vi "Main.vi"(10 "DAQ Type":enum16{"Hardware", "Simulation"}(ring), 11 "Module Admin":refnum<class "Delacor_lib_QMH_Module Admin.lvclass">) -> ()   [LabVIEW 2021, in "DAQ IO.lvlib"]
doc: "This template is based off of the Queued Message Handler design pattern and the Queued Message Handler project template that ships with LabVIEW.\n\nThe main difference is that the queue is private to this module and communication between modules is performed via Broadcast and Request events.\n\nRequest events are wrapped in public API methods and are handled in the Event Handling Loop (EHL) of this VI. Any module can register for Broadcast events sent by this module. The EHL generates messages based on user interface actions.\n\nThe Message Handling Loop (MHL) processes messages generated by the EHL, or by other messages. The messages are string values, so new messages can be added easily to the Message Cases case structure in the MHL. Each message cluster can also provide an optional value for Message Data, which is a variant that can be converted to whatever message-specific data is required.\n_____\nBased on DQMH Project Template 6.1.0.94."
uses:
  DAQ IO.lvlib
  <vilib>/Delacor/Delacor QMH/Libraries/Message Queue_class/Delacor_lib_QMH_Message Queue.lvclass
  Module Data--cluster.ctl
  <vilib>/Utility/miscctls.llb/LVPointTypeDef.ctl
  <vilib>/Utility/error.llb/Error Cluster From Error Code.vi
  <vilib>/ErrorRing/Error Ring.xnode
  <vilib>/Delacor/Delacor QMH/Libraries/Message Queue_class/Delacor_lib_QMH_Enqueue Message (Single).vi
  Stop Argument--cluster.ctl
  <vilib>/Delacor/Delacor QMH/Libraries/Module Admin_class/Delacor_lib_QMH_Module Admin.lvclass
  REQ Initialize DI (Reply Payload)--cluster.ctl
  REQ Initialize DI Argument--cluster.ctl
  Class/Abstract/Abstract.lvclass
  Class/PXI 6515/PXI 6515.lvclass
  REQ Initialize DO (Reply Payload)--cluster.ctl
  REQ Initialize DO Argument--cluster.ctl
  DO Name.ctl
  REQ Write DO Argument--cluster.ctl
  REQ Close DI Argument--cluster.ctl
  REQ Close DO Argument--cluster.ctl
  DI Channel Setting.ctl
  DO Channel Setting.ctl
  REQ Acq DI Argument--cluster.ctl
  C:/repository/common_ATE/Libraries/DAQ IO/Class/Abstract/Abstract.lvclass
  C:/repository/common_ATE/Libraries/DAQ IO/Class/PXI 6515/PXI 6515.lvclass
panel:
  out "DO  Setting":T1
  out "DI  Setting":T2
  in  "Acquire DI ?":bool
  out "error out":errorcluster
  out "Status":string
  in  "Simulate MHL Error":bool
  in  "Simulate EHL Error":bool
  # "Other QMH Modules communicate with this Module via its Public API (wrappers for its Request Events).\n\nThis Module communicates with other Modules via its Broadcast Events.\nAny module that wants to get these messages, just registers for this module's Broadcast events."
  # "This template is for the Delacor Modified Queued Message Handler design pattern.\n\nSee the block diagram for more information on how to use this template."
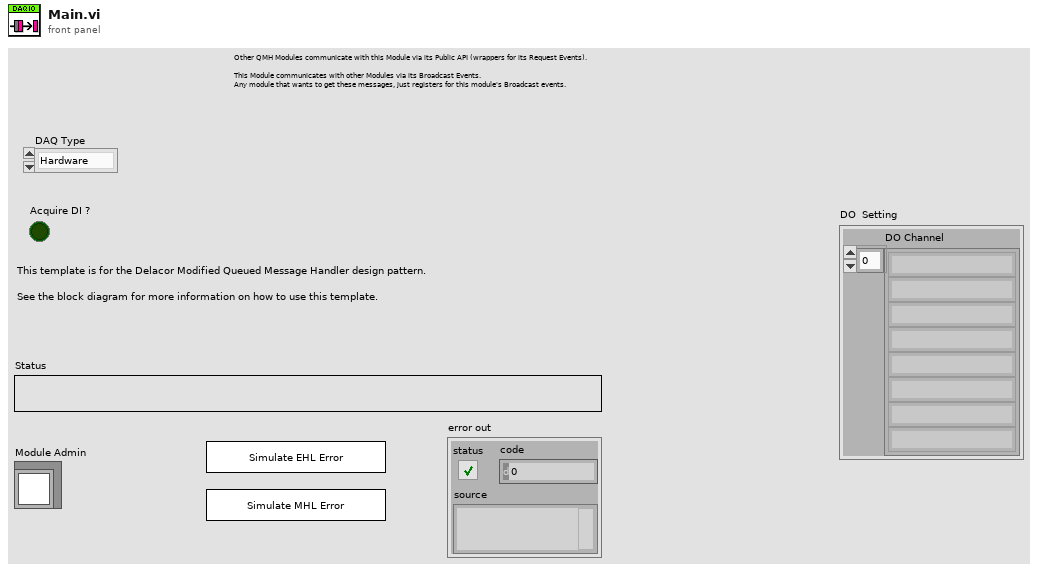
[diagram p1: front panel]
types:
  T1 = typedef "DAQ IO.lvlib/DO Channel Setting.ctl" = cluster{"DO Channel":string[]}
  T2 = typedef "DAQ IO.lvlib/DI Channel Setting.ctl" = cluster{"DI Channel":string[]}
  T3 = typedef "DAQ IO.lvlib/Module Data--cluster.ctl" = cluster{"Status":string, "Abstract.lvclass":refnum<class "Abstract.lvclass">, "DI Channel Setting":T2}
  T4 = typedef "DAQ IO.lvlib/Request Events--cluster.ctl" = cluster{"Stop Module":refnum<user-event>, "Show Panel":refnum<user-event>, "Hide Panel":refnum<user-event>, "Get Module Execution Status":refnum<user-event>, "Show Diagram":refnum<user-event>, "REQ Initialize DI":refnum<user-event>, "REQ Initialize DO":refnum<user-event>, "REQ Write DO":refnum<user-event>, "REQ Close DI":refnum<user-event>, "REQ Close DO":refnum<user-event>, "REQ Acq DI":refnum<user-event>}
  T5 = enum32{"invalid lock state", "Not Locked", "Locked (No Password)", "Password-protected"}
  T6 = typedef "DAQ IO.lvlib/Stop Argument--cluster.ctl" = cluster{"Origin":string, "Exit via Stop Module Req?":bool, "Wait for Module to stop?":bool}
  T7 = typedef "DAQ IO.lvlib/REQ Initialize DI Argument--cluster.ctl" = cluster{"Wait Notifier":refnum<notifier>, "wait for reply":bool, "DI Channel Setting":T2}
  T8 = typedef "DAQ IO.lvlib/REQ Initialize DO Argument--cluster.ctl" = cluster{"Wait Notifier":refnum<notifier>, "wait for reply":bool, "DO Channel Setting":T1}
  T9 = typedef "DAQ IO.lvlib/REQ Write DO Argument--cluster.ctl" = cluster{"DO Name":T10, "DO Value":bool[]}
  T10 = typedef "DAQ IO.lvlib/DO Name.ctl" = enum16{"Emg", "Start", "Stop", "Retry"}
  T11 = typedef "DAQ IO.lvlib/REQ Close DI Argument--cluster.ctl" = cluster{"Boolean":bool}
  T12 = typedef "DAQ IO.lvlib/REQ Close DO Argument--cluster.ctl" = cluster{"Boolean":bool}
  T13 = typedef "DAQ IO.lvlib/REQ Acq DI Argument--cluster.ctl" = cluster{"Acq DI":bool}
  T14 = typedef "LVPointTypeDef.ctl" = cluster{"Horizontal":i16, "Vertical":i16}
  T15 = enum32{"Invalid", "Standard", "Closed", "Hidden", "Minimized", "Maximized"}
  T16 = typedef "DAQ IO.lvlib/REQ Initialize DI (Reply Payload)--cluster.ctl" = cluster{"Connect?":bool, "error":errorcluster}
  T17 = typedef "DAQ IO.lvlib/REQ Initialize DO (Reply Payload)--cluster.ctl" = cluster{"Connect?":bool, "error":errorcluster}
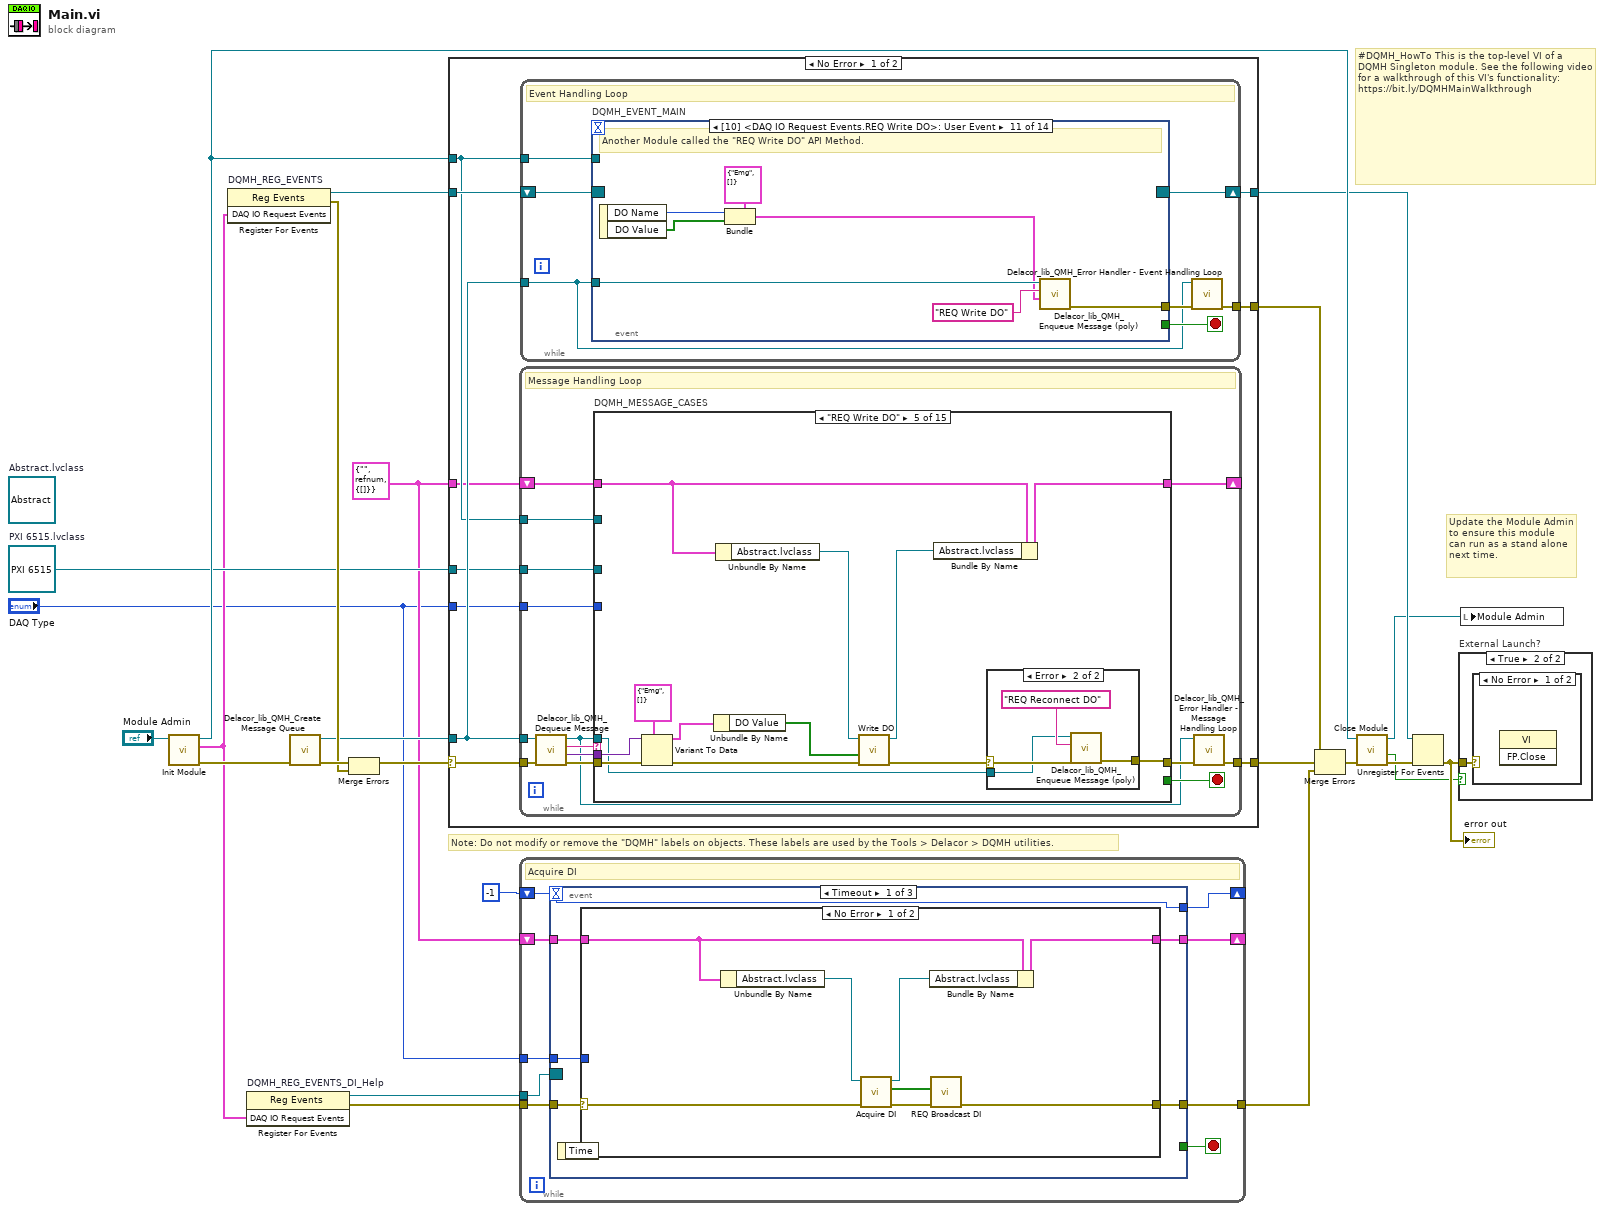
[diagram p0: block diagram]
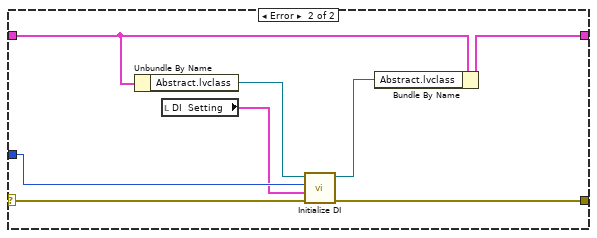
[diagram p2: hidden frame]
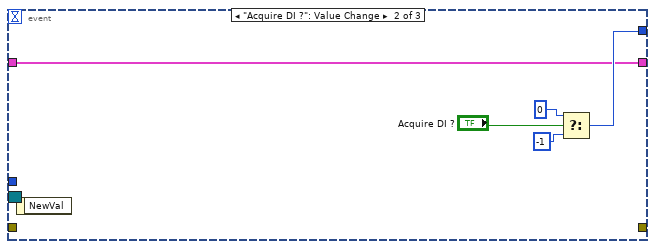
[diagram p3: hidden frame]
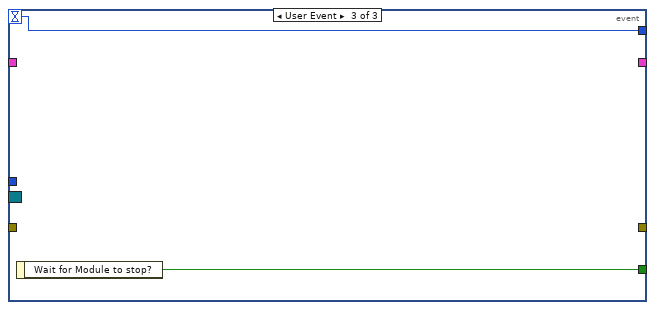
[diagram p4: hidden frame]
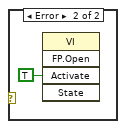
[diagram p6: hidden frame]
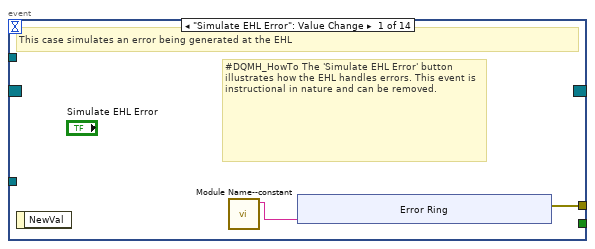
[diagram p7: hidden frame]
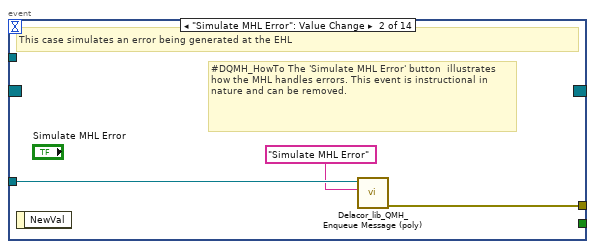
[diagram p8: hidden frame]
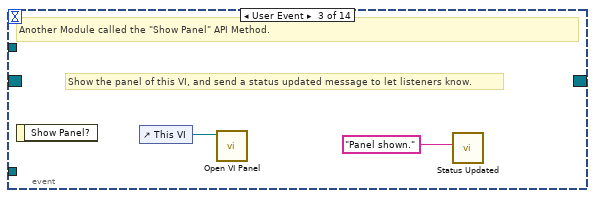
[diagram p9: hidden frame]
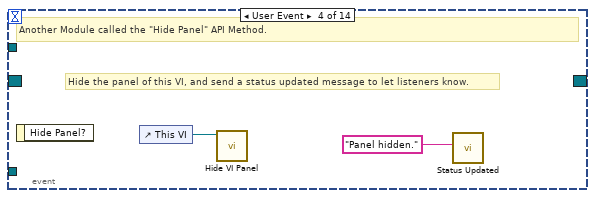
[diagram p10: hidden frame]
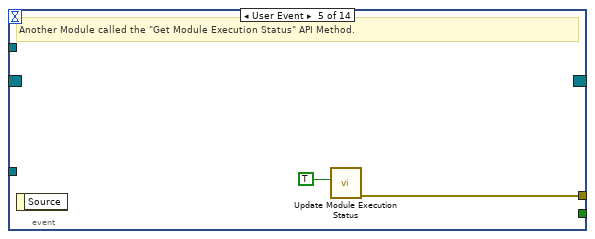
[diagram p11: hidden frame]
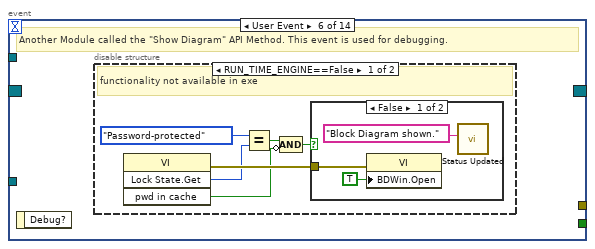
[diagram p12: hidden frame]
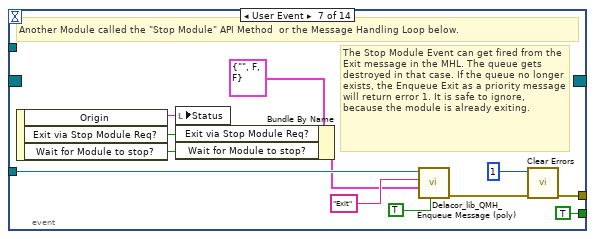
[diagram p15: hidden frame]
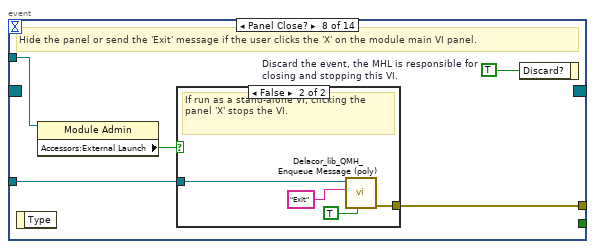
[diagram p16: hidden frame]
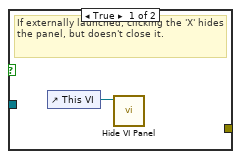
[diagram p17: hidden frame]
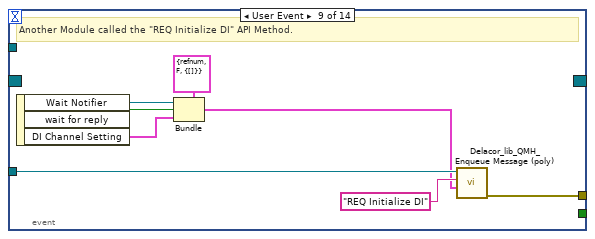
[diagram p18: hidden frame]
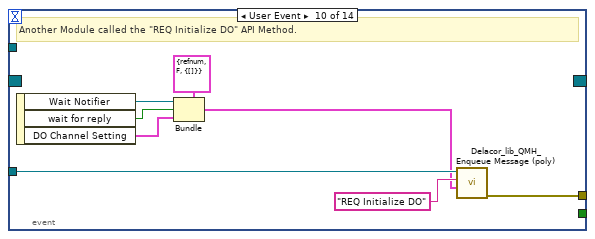
[diagram p19: hidden frame]
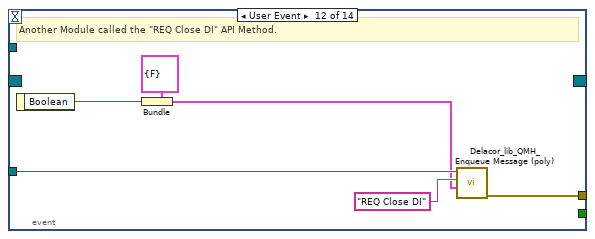
[diagram p20: hidden frame]
diagram:
  w4 = T3 {"Status"="", "Abstract.lvclass"=refnum, "DI Channel Setting"={"DI Channel"=[]}} ("Data Cluster")
  w9 = refnum<class "PXI 6515.lvclass"> refnum  # PXI 6515.lvclass
  (unwired) refnum<class "Abstract.lvclass"> refnum  # Abstract.lvclass
  # "#DQMH_HowTo This is the top-level VI of a DQMH Singleton module. See the following video for a walkthrough of this VI's functionality: https://bit.ly/DQMHMainWalkthrough"
  # "Note: Do not modify or remove the \"DQMH\" labels on objects. These labels are used by the Tools > Delacor > DQMH utilities."
  # "Update the Module Admin to ensure this module can run as a stand alone next time."
  n1 = call "Init Module.vi"("Singleton Module Admin in"="Module Admin") -> ("error out"=w23:errorcluster, "DAQ IO Request Events"=w8:T4, "Singleton Module Admin out"=w16:refnum<class "Delacor_lib_QMH_Module Admin.lvclass">)  [unwired: 8 in]
  n2 = register-events "DQMH_REG_EVENTS"(w8) -> (reference out=w14:refnum<event-registration>, error out=w17:errorcluster)  [unwired: 2 in]
  n3 = register-events "DQMH_REG_EVENTS_DI_Help"(w8) -> (reference out=w7:refnum<event-registration>, error out=w6:errorcluster)  [unwired: 2 in]
  n4 = call <vilib>:"Delacor_lib_QMH_Create Message Queue.vi"("error in"=w23) -> ("error out"=w19:errorcluster, "Message Queue"=w13:refnum<class "Delacor_lib_QMH_Message Queue.lvclass">)  [unwired: 9 in]
  n5 = Merge Errors(w19, w17) -> (w18:errorcluster)
  n6 = case shown="No Error" w18 {
    selector: w18 -> [w32 w327]
    tunnel: [w34 w326] -> w24
    tunnel: [w31 w332] -> w15
    tunnel: w14 -> [w30 w332]
    tunnel: w13 -> [w29 w325]
    tunnel: [w33 _] -> w3
    tunnel: w16 -> [w28 w328]
    tunnel: w9 -> [w27 _]
    tunnel: "DAQ Type" -> [w26 _]
    tunnel: w4 -> [w25 _]
    frame No Error {
      n7 = while {
        tunnel: w29 -> [w136]
        shift-right: [w140] -> _
        shift-left: w25 -> [w141]
        tunnel: w32 -> [w144]
        tunnel: [w142] -> w34
        tunnel: w28 -> [w134]
        tunnel: w27 -> [w133]
        tunnel: w26 -> [w132]
        stop <- w139 stop-if-true
        # "Message Handling Loop"
        n8 = call-dynamic "Delacor_lib_QMH_Dequeue Message.vi"("error in"=w144, "Message Queue in"=w136) -> ("error out"=w143:errorcluster, "Message Data"=w137:variant, "Message"=w138:string, "Message Queue out"=w135:refnum<class "Delacor_lib_QMH_Message Queue.lvclass">)  [unwired: 6 in]
        n9 = case "DQMH_MESSAGE_CASES" shown="\"REQ Write DO\"" w138 {
          selector: w138 -> [_ _ _ _ _ _ _ _ _ _ _ _ _ _ w312]
          tunnel: w135 -> [_ _ _ _ w209 _ _ w251 _ _ _ _ w282 w304 _]
          tunnel: w143 -> [w164 w168 w186 w206 w221 w236 w246 w253 w262 w265 w267 w272 w289 w310 w314]
          tunnel: [w162 w168 w175 w195 w210 w231 w241 w252 w255 w264 w267 w271 w285 w307 w315] -> w145
          tunnel: w141 -> [w153 w167 w172 w191 w216 w230 w240 w254 w261 w263 w266 w269 w284 w303 w313]
          tunnel: [w152 w167 w176 w197 w214 w228 w238 w254 w261 w263 w266 w269 w284 w303 w313] -> w140
          tunnel: [_ _ _ _ _ _ _ _ _ _ _ _ _ w302 _] -> w139
          tunnel: w137 -> [_ _ w185 w205 w220 w235 w245 _ w260 _ _ _ w283 w301 _]
          tunnel: w134 -> [w154 _ _ _ _ _ _ _ _ _ _ _ w281 w296 _]
          tunnel: w133 -> [w146 _ _ _ _ _ _ _ _ _ _ _ _ _ _]
          tunnel: w132 -> [_ _ w177 w192 _ _ _ _ _ _ _ _ _ _ _]
          frame "Initialize" {
            w148 = "Initial Message" ("Initial Message")
            # "Initialize - Any operation that needs to be done before the module can receive messages. Synchronize Caller Events.vi will inform Start Module.vi that the module has launched and is ready to receive messages. Module Did Init.vi will broadcast that the module initialized."
            n10 = call "Synchronize Caller Events.vi"("error in (no error)"=w164, "Singleton Module Admin in"=w154) -> ("error out"=w163:errorcluster, "Singleton Module Admin out"=w149:refnum<class "Delacor_lib_QMH_Module Admin.lvclass">)  [unwired: 8 in]
            n11 = property class="Module Admin"(reference=w149) -> ("Accessors:External Launch"=w158:bool)  [unwired: 1 in, 2 out]
            n12 = Select(t=T15."Hidden" ("State"), s=w158, f=T15."Standard" ("State")) -> (s? t:f=w155:T15)
            n13 = call "Module Name--constant.vi"() -> ("Module Name"=w161:string)  [unwired: 11 in]
            n14 = property class="VI"("Front Panel.Title"=w161) -> (reference out=w160:refnum<vi>, error out=w166:errorcluster)  [unwired: 2 in]
            n15 = call "Module Name--constant.vi"() -> ("Module Name"=w150:string)  [unwired: 11 in]
            n16 = Bundle By Name(cluster=w153, "Status"=w148, "Abstract.lvclass"=w146) -> (w152:T3)
            n17 = invoke class="VI" method="FP.Open"(reference=w160, error in=w166, "State"=w155) -> (reference out=w159:refnum<vi>, error out=w165:errorcluster)  [unwired: 2 in, 3 out]
            n18 = call "Module Did Init.vi"("error in (no error)"=w163, "Initialized?"=TRUE, "Origin"=w150) -> ("error out"=w162:errorcluster)  [unwired: 8 in]
            n19 = invoke class="VI" method="FP.Center"(reference=w159, error in=w165) -> ()  [unwired: 1 in, 3 out]
            n20 = property on="Pane" class="Pane"("Origin"=T14 {"Horizontal"=0, "Vertical"=0}) -> ()  [unwired: 2 in, 2 out]
            "Status" <- w148
          }
          frame "---Module Specific---" {
            # "Separator -- The following cases handle messages specific to this Module."
          }
          frame "REQ Initialize DI" {
            n21 = Variant To Data(error in=w186, type=T7 {"Wait Notifier"=refnum, "wait for reply"=FALSE, "DI Channel Setting"={"DI Channel"=[]}} ("REQ Initialize DI Argument"), Variant=w185) -> (data=w183:T7, error out=w178:errorcluster)
            n22 = Unbundle By Name(w183) -> ("Wait Notifier"=w182:refnum<notifier>, "wait for reply"=w181:bool, "DI Channel Setting"=w169:T2)
            "DI  Setting" <- w169
            n23 = Unbundle By Name(w172) -> ("Abstract.lvclass"=w171:refnum<class "Abstract.lvclass">)
            n24 = call-dynamic "Initialize DI.vi"("error in (no error)"=w178, "DI Channel Setting"=w169, "DAQ Type"=w177, "Abstract in"=w171) -> ("error out"=w175:errorcluster, "Abstract out"=w170:refnum<class "Abstract.lvclass">)  [unwired: 6 in]
            n25 = Unbundle By Name(w175) -> ("status"=w174:bool)
            n26 = Bundle By Name(cluster=w172, "Abstract.lvclass"=w170) -> (w176:T3)
            n27 = Not(x=w174) -> (.not. x?=w173:bool)
            n28 = Bundle By Name(cluster=T16 {"Connect?"=FALSE, "error"={"status"=FALSE, "code"=0, "source"=""}} ("REQ Initialize DI (Reply Payload)"), "Connect?"=w173) -> (w180:T16)
            n29 = case shown="True" w181 {
              tunnel: w182 -> [_ w188]
              tunnel: w180 -> [_ w187]
              frame False {
              }
              frame True {
                n30 = Send Notification(notification=w187, notifier=w188) -> ()  [unwired: 1 in, 2 out]
              }
            }
          }
          frame "REQ Initialize DO" {
            n31 = Variant To Data(error in=w206, type=T8 {"Wait Notifier"=refnum, "wait for reply"=FALSE, "DO Channel Setting"={"DO Channel"=[]}} ("REQ Initialize DO Argument"), Variant=w205) -> (data=w203:T8, error out=w198:errorcluster)
            n32 = Unbundle By Name(w191) -> ("Abstract.lvclass"=w190:refnum<class "Abstract.lvclass">)
            n33 = Unbundle By Name(w203) -> ("Wait Notifier"=w202:refnum<notifier>, "wait for reply"=w201:bool, "DO Channel Setting"=w189:T1)
            "DO  Setting" <- w189
            n34 = call-dynamic "Initialize DO.vi"("error in (no error)"=w198, "DO Channel Setting"=w189, "DAQ Type"=w192, "Abstract in"=w190) -> ("error out"=w195:errorcluster, "Abstract out"=w196:refnum<class "Abstract.lvclass">)  [unwired: 6 in]
            n35 = Unbundle By Name(w195) -> ("status"=w194:bool)
            n36 = Bundle By Name(cluster=w191, "Abstract.lvclass"=w196) -> (w197:T3)
            n37 = Not(x=w194) -> (.not. x?=w193:bool)
            n38 = Bundle By Name(cluster=T17 {"Connect?"=FALSE, "error"={"status"=FALSE, "code"=0, "source"=""}} ("REQ Initialize DO (Reply Payload)"), "Connect?"=w193) -> (w200:T17)
            n39 = case shown="True" w201 {
              tunnel: w202 -> [_ w208]
              tunnel: w200 -> [_ w207]
              frame False {
              }
              frame True {
                n40 = Send Notification(notification=w207, notifier=w208) -> ()  [unwired: 1 in, 2 out]
              }
            }
          }
          frame "REQ Write DO" {
            n41 = Variant To Data(error in=w221, type=T9 {"DO Name"=enum."Emg", "DO Value"=[]} ("REQ Write DO Argument"), Variant=w220) -> (data=w218:T9, error out=w217:errorcluster)
            n42 = Unbundle By Name(w218) -> ("DO Value"=w212:bool[])
            n43 = Unbundle By Name(w216) -> ("Abstract.lvclass"=w215:refnum<class "Abstract.lvclass">)
            n44 = call-dynamic "Write DO.vi"("error in (no error)"=w217, "DO Value"=w212, "Abstract in"=w215) -> ("error out"=w211:errorcluster, "Abstract out"=w213:refnum<class "Abstract.lvclass">)  [unwired: 7 in]
            n45 = Bundle By Name(cluster=w216, "Abstract.lvclass"=w213) -> (w214:T3)
            n46 = case shown="Error" w211 {
              selector: w211 -> [w222 w225]
              tunnel: [w222 w224] -> w210
              tunnel: w209 -> [_ w223]
              frame No Error {
              }
              frame Error {
                n47 = call-poly <vilib>:"Delacor_lib_QMH_Enqueue Message (poly).vi"("error in"=w225, "Message"="REQ Reconnect DO", "Message Queue in"=w223) -> ("error out"=w224:errorcluster)  [unwired: 7 in, 1 out]
              }
            }
          }
          frame "REQ Close DI" {
            n48 = Variant To Data(error in=w236, type=T11 {"Boolean"=FALSE} ("REQ Close DI Argument"), Variant=w235) -> (data=w233:T11, error out=w232:errorcluster)
            n49 = Unbundle By Name(w233) -> ()  [unwired: 1 out]
            n50 = Unbundle By Name(w230) -> ("Abstract.lvclass"=w229:refnum<class "Abstract.lvclass">)
            n51 = call-dynamic "Close DI Ref.vi"("error in (no error)"=w232, "Abstract in"=w229) -> ("error out"=w231:errorcluster, "Abstract out"=w227:refnum<class "Abstract.lvclass">)  [unwired: 8 in]
            n52 = Bundle By Name(cluster=w230, "Abstract.lvclass"=w227) -> (w228:T3)
          }
          frame "REQ Close DO" {
            n53 = Variant To Data(error in=w246, type=T12 {"Boolean"=FALSE} ("REQ Close DO Argument"), Variant=w245) -> (data=w243:T12, error out=w242:errorcluster)
            n54 = Unbundle By Name(w243) -> ()  [unwired: 1 out]
            n55 = Unbundle By Name(w240) -> ("Abstract.lvclass"=w239:refnum<class "Abstract.lvclass">)
            n56 = call-dynamic "Close DO Ref.vi"("error in (no error)"=w242, "Abstract in"=w239) -> ("error out"=w241:errorcluster, "Abstract out"=w237:refnum<class "Abstract.lvclass">)  [unwired: 8 in]
            n57 = Bundle By Name(cluster=w240, "Abstract.lvclass"=w237) -> (w238:T3)
          }
          frame "REQ Reconnect DO" {
            # "Duplicate this frame when creating new messages.  Change this comment in the duplicated frame to describe this message."
            n58 = local read "DO  Setting"() -> (w248:T1)
            n59 = Bundle By Name(cluster=T8 {"Wait Notifier"=refnum, "wait for reply"=FALSE, "DO Channel Setting"={"DO Channel"=[]}} ("REQ Initialize DO Argument"), "DO Channel Setting"=w248) -> (w247:T8)
            n60 = call-poly <vilib>:"Delacor_lib_QMH_Enqueue Message (poly).vi"("error in"=w253, "Message Data"=w247, "Message"="REQ Initialize DO" ("String"), "Message Queue in"=w251) -> ("error out"=w252:errorcluster)  [unwired: 6 in, 1 out]
          }
          frame "REQ Acq DI" {
            n61 = Variant To Data(error in=w262, type=T13 {"Acq DI"=FALSE} ("REQ Acq DI Argument"), Variant=w260) -> (data=w258:T13, error out=w257:errorcluster)
            n62 = Unbundle By Name(w258) -> ("Acq DI"=w256:bool)
            n63 = property on="Acquire DI ?" class="Bool (strict)"(error in=w257, "Val(Sgnl)"=w256) -> (error out=w255:errorcluster)  [unwired: 1 in, 1 out]
          }
          frame "---Copy This Frame---" {
            # "Duplicate this frame when creating new messages.  Change this comment in the duplicated frame to describe this message."
            n64 = Merge Errors(w265) -> (w264:errorcluster)
          }
          frame "---Exit and Error Handling---" {
            # "Separator - The following cases handle errors and exit messages."
          }
          frame "Simulate MHL Error" {
            # "#DQMH_HowTo The 'Simulate MHL Error' button  illustrates how the MHL handles errors. This event is instructional in nature and can be removed."
            # "Simulate an error occurring at the MHL"
            n65 = call "Module Name--constant.vi"() -> ("Module Name"=w268:string)  [unwired: 11 in]
            n66 = xnode "Error Ring"("parameter 0"=w268) -> ("error out"=w270:errorcluster)
            n67 = Merge Errors(w272, w270) -> (w271:errorcluster)
          }
          frame "Error" {
            # "#CodeRecommended - If you ever change the name of this \"Error\" message, you'll need to update the name in the Check Loop Error.vi as well."
            # "#CodeRecommended - If the module is running in standalone mode (External Launch = FALSE), this code will pop up an error dialog and call the 'Exit' message if an error occurs. Add more fine-grained error handling here."
            # "Error - Check the error message data and respond accordingly. This message is sent by the \"Error Handler\" VIs at the end of each loop in this application."
            n68 = property class="Module Admin"(reference=w281) -> ("Accessors:External Launch"=w280:bool)  [unwired: 1 in, 2 out]
            n69 = Variant To Data(error in=w289, type=errorcluster {"status"=FALSE, "code"=0, "source"=""} ("error constant"), Variant=w283) -> (data=w290:errorcluster, error out=w287:errorcluster)
            n70 = call "Error Reported.vi"("Error"=w290) -> ()  [unwired: 10 in, 1 out]
            n71 = case shown="False" w280 {
              tunnel: [w295 _] -> w286
              tunnel: w282 -> [w293 _]
              tunnel: w290 -> [w294 _]
              frame False {
                (unwired) "Exit"
                n72 = call <vilib>:"Simple Error Handler.vi"("error in (no error)"=w294) -> ()  [unwired: 4 in, 5 out]
                n73 = call-poly <vilib>:"Delacor_lib_QMH_Enqueue Message (poly).vi"("Priority Message? (F)"=TRUE, "Message"="REQ Reconnect", "Message Queue in"=w293) -> ("error out"=w295:errorcluster)  [unwired: 7 in, 1 out]
              }
              frame True {
                # "If the module was launched externally, calling the Error Reported broadcast VI is the only action performed by the \"Error\" message. The module's caller can then process the error appropriately."
              }
            }
            n74 = Merge Errors(w287, w286) -> (w285:errorcluster)
            n75 = local write "error out"(w285) -> ()
          }
          frame "Exit" {
            w300 = 91  # 91: not all Exit messages will have an argument
            w302 = TRUE  # Stop the VI
            # "Release the message queue reference"
            # "#CodeNeeded - Add any required cleanup code here"
            # "Exit - Exit the application."
            n76 = Variant To Data(error in=w310, type=T6 {"Origin"="", "Exit via Stop Module Req?"=FALSE, "Wait for Module to stop?"=FALSE} ("Stop Argument"), Variant=w301) -> (data=w298:T6, error out=w306:errorcluster)
            n77 = call <vilib>:"Clear Errors.vi"("error in (no error)"=w306, "specific error code to clear (0: all)"=w300) -> ("error out"=w309:errorcluster)  [unwired: 4 in, 1 out]
            n78 = control-ref of="This VI"() -> (w297:refnum<vi>)
            n79 = call-dynamic "Delacor_lib_QMH_Release Message Queue.vi"("error in"=w309, "Message Queue"=w304) -> ("error out"=w308:errorcluster)  [unwired: 9 in]
            n80 = call "Handle Exit.vi"("Stop Argument"=w298, "Admin in"=w296, "VI reference"=w297) -> ("error out"=w305:errorcluster)  [unwired: 7 in, 1 out]
            n81 = Merge Errors(w308, w305) -> (w307:errorcluster)
          }
          frame Default {
            # "'Default' case only runs if there is a message that isn't defined in any of the other cases.  Output a programming error."
            n82 = call "Module Name--constant.vi"() -> ("Module Name"=w311:string)  [unwired: 11 in]
            n83 = xnode "Error Ring"("parameter 0"=w312, "parameter 1"=w311) -> ("error out"=w316:errorcluster)
            n84 = Merge Errors(w314, w316) -> (w315:errorcluster)
          }
        }
        n85 = call-dynamic "Delacor_lib_QMH_Error Handler - Message Handling Loop.vi"("error in"=w145, "Message Queue in"=w135) -> ("dup error in"=w142:errorcluster)  [unwired: 8 in, 1 out]
      }
      n86 = while {
        tunnel: w29 -> [w35]
        shift-right: [w38] -> w31
        shift-left: w30 -> [w39]
        tunnel: [w40] -> w33
        tunnel: w28 -> [w36]
        stop <- w37 stop-if-true
        # "Event Handling Loop"
        n87 = event "DQMH_EVENT_MAIN" shown="[10] <DAQ IO Request Events.REQ Write DO>: User Event" {
          selector: w39 -> [_ _ _ _ _ _ _ _ _ _ _ _ _ _]
          dyn-events: [_ _ _ _ _ _ _ _ _ _ _ _ _ _] -> w38
          timeout: _ -> [_ _ _ _ _ _ _ _ _ _ _ _ _ _]
          tunnel: [_ _ _ _ _ _ TRUE ("Discard?") _ _ _ _ _ _ _] -> w37
          tunnel: w35 -> [_ w52 _ _ _ _ w76 w83 w98 w106 w113 w119 w125 w131]
          tunnel: [w43 w53 _ _ w59 _ w79 w85 w94 w100 w107 w114 w120 w126] -> w41
          tunnel: w36 -> [_ _ _ _ _ _ _ w82 _ _ _ _ _ _]
          event "Simulate EHL Error": Value Change {
            # "#DQMH_HowTo The 'Simulate EHL Error' button  illustrates how the EHL handles errors. This event is instructional in nature and can be removed."
            # "This case simulates an error being generated at the EHL"
            n88 = event-data() -> ()  [unwired: 1 in, 1 out]
            n89 = call "Module Name--constant.vi"() -> ("Module Name"=w42:string)  [unwired: 11 in]
            n90 = xnode "Error Ring"("parameter 0"=w42) -> ("error out"=w43:errorcluster)
          }
          event "Simulate MHL Error": Value Change {
            # "#DQMH_HowTo The 'Simulate MHL Error' button  illustrates how the MHL handles errors. This event is instructional in nature and can be removed."
            # "This case simulates an error being generated at the EHL"
            n91 = event-data() -> ()  [unwired: 1 in, 1 out]
            n92 = call-poly <vilib>:"Delacor_lib_QMH_Enqueue Message (poly).vi"("Message"="Simulate MHL Error", "Message Queue in"=w52) -> ("error out"=w53:errorcluster)  [unwired: 8 in, 1 out]
          }
          event User Event {
            # "Show the panel of this VI, and send a status updated message to let listeners know."
            # "Another Module called the \"Show Panel\" API Method."
            n93 = event-data() -> ()  [unwired: 1 in, 1 out]
            n94 = control-ref of="This VI"() -> (w55:refnum<vi>)
            n95 = call "Open VI Panel.vi"("VI"=w55) -> ()  [unwired: 10 in, 1 out]
            n96 = call "Status Updated.vi"("Status"="Panel shown." ("format string")) -> ()  [unwired: 10 in, 1 out]
          }
          event User Event {
            # "Hide the panel of this VI, and send a status updated message to let listeners know."
            # "Another Module called the \"Hide Panel\" API Method."
            n97 = event-data() -> ()  [unwired: 1 in, 1 out]
            n98 = control-ref of="This VI"() -> (w57:refnum<vi>)
            n99 = call "Hide VI Panel.vi"("VI"=w57) -> ()  [unwired: 10 in, 1 out]
            n100 = call "Status Updated.vi"("Status"="Panel hidden." ("format string")) -> ()  [unwired: 10 in, 1 out]
          }
          event User Event {
            # "Another Module called the \"Get Module Execution Status\" API Method."
            n101 = event-data() -> ()  [unwired: 1 in, 1 out]
            n102 = call "Update Module Execution Status.vi"("Running?"=TRUE) -> ("error out"=w59:errorcluster)  [unwired: 10 in]
          }
          event User Event {
            # "Another Module called the \"Show Diagram\" API Method. This event is used for debugging."
            n103 = event-data() -> ()  [unwired: 1 in, 1 out]
            n104 = disable-structure shown="RUN_TIME_ENGINE==False" {
              frame condition #0 (active) {
                # "functionality not available in exe"
                n105 = invoke class="VI" method="Lock State.Get"() -> (error out=w65:errorcluster, "Get Lock State"=w64:T5, "pwd in cache"=w61:bool)  [unwired: 4 in, 1 out]
                n106 = Equal?(x=T5."Password-protected", y=w64) -> (x = y?=w62:bool)
                n107 = Compound Arithmetic op=AND(w62, invert w61) -> (w60:bool)
                n108 = case shown="False" w60 {
                  tunnel: w65 -> [w68 _]
                  frame False {
                    n109 = property class="VI"(error in=w68, "BDWin.Open"=TRUE ("Block Diagram Window:Open")) -> ()  [unwired: 1 in, 2 out]
                    n110 = call "Status Updated.vi"("Status"="Block Diagram shown." ("format string")) -> ()  [unwired: 10 in, 1 out]
                  }
                  frame True {
                    # "Password-protected VI, and the password is not in the cache. Do not show the diagram."
                  }
                }
              }
              frame condition #1 {
              }
            }
          }
          event User Event {
            # "The Stop Module Event can get fired from the Exit message in the MHL. The queue gets destroyed in that case. If the queue no longer exists, the Enqueue Exit as a priority message will return error 1. It is safe to ignore, because the module is already exiting."
            # "Another Module called the \"Stop Module\" API Method  or the Message Handling Loop below."
            n111 = event-data() -> ("Origin"=w75:string, "Exit via Stop Module Req?"=w71:bool, "Wait for Module to stop?"=w70:bool)  [unwired: 1 in]
            n112 = local write "Status"(w75) -> ()
            n113 = Bundle By Name(cluster=T6 {"Origin"="", "Exit via Stop Module Req?"=FALSE, "Wait for Module to stop?"=FALSE} ("Stop Argument"), "Exit via Stop Module Req?"=w71, "Wait for Module to stop?"=w70) -> (w69:T6)
            n114 = call-poly <vilib>:"Delacor_lib_QMH_Enqueue Message (poly).vi"("Priority Message? (F)"=TRUE, "Message Data"=w69, "Message"="Exit", "Message Queue in"=w76) -> ("error out"=w80:errorcluster)  [unwired: 6 in, 1 out]
            n115 = call <vilib>:"Clear Errors.vi"("error in (no error)"=w80, "specific error code to clear (0: all)"=1) -> ("error out"=w79:errorcluster)  [unwired: 4 in, 1 out]
          }
          event Panel Close? {
            w84 = TRUE  # Discard the event, the MHL is responsible for closing and stopping this VI.
            # "Hide the panel or send the 'Exit' message if the user clicks the 'X' on the module main VI panel."
            n116 = event-data() -> ()  [unwired: 1 in, 1 out]
            n117 = property class="Module Admin"(reference=w82) -> ("Accessors:External Launch"=w81:bool)  [unwired: 1 in, 2 out]
            n118 = case shown="False" w81 {
              tunnel: w83 -> [_ w89]
              tunnel: [_ w90] -> w85
              frame True {
                # "If externally launched, clicking the 'X' hides the panel, but doesn't close it."
                n119 = control-ref of="This VI"() -> (w86:refnum<vi>)
                n120 = call "Hide VI Panel.vi"("VI"=w86) -> ()  [unwired: 10 in, 1 out]
              }
              frame False {
                # "If run as a stand-alone VI, clicking the panel 'X' stops the VI."
                n121 = call-poly <vilib>:"Delacor_lib_QMH_Enqueue Message (poly).vi"("Priority Message? (F)"=TRUE, "Message"="Exit", "Message Queue in"=w89) -> ("error out"=w90:errorcluster)  [unwired: 7 in, 1 out]
              }
            }
            n122 = event-data("Discard?"=w84) -> ()  [unwired: 1 in, 1 out]
          }
          event User Event {
            # "Another Module called the \"REQ Initialize DI\" API Method."
            n123 = event-data() -> ("Wait Notifier"=w93:refnum<notifier>, "wait for reply"=w92:bool, "DI Channel Setting"=w91:T2)  [unwired: 1 in]
            n124 = Bundle(cluster=T7 {"Wait Notifier"=refnum, "wait for reply"=FALSE, "DI Channel Setting"={"DI Channel"=[]}} ("REQ Initialize DI Argument"), "Wait Notifier"=w93, "wait for reply"=w92, "DI Channel Setting"=w91) -> (w95:T7)
            n125 = call-poly <vilib>:"Delacor_lib_QMH_Enqueue Message (poly).vi"("Message Data"=w95, "Message"="REQ Initialize DI", "Message Queue in"=w98) -> ("error out"=w94:errorcluster)  [unwired: 7 in, 1 out]
          }
          event User Event {
            # "Another Module called the \"REQ Initialize DO\" API Method."
            n126 = event-data() -> ("Wait Notifier"=w102:refnum<notifier>, "wait for reply"=w101:bool, "DO Channel Setting"=w99:T1)  [unwired: 1 in]
            n127 = Bundle(cluster=T8 {"Wait Notifier"=refnum, "wait for reply"=FALSE, "DO Channel Setting"={"DO Channel"=[]}} ("REQ Initialize DO Argument"), "Wait Notifier"=w102, "wait for reply"=w101, "DO Channel Setting"=w99) -> (w103:T8)
            n128 = call-poly <vilib>:"Delacor_lib_QMH_Enqueue Message (poly).vi"("Message Data"=w103, "Message"="REQ Initialize DO", "Message Queue in"=w106) -> ("error out"=w100:errorcluster)  [unwired: 7 in, 1 out]
          }
          event User Event {
            # "Another Module called the \"REQ Write DO\" API Method."
            n129 = event-data() -> ("DO Name"=w109:T10, "DO Value"=w108:bool[])  [unwired: 1 in]
            n130 = Bundle(cluster=T9 {"DO Name"=enum."Emg", "DO Value"=[]} ("REQ Write DO Argument"), "DO Name"=w109, "DO Value"=w108) -> (w110:T9)
            n131 = call-poly <vilib>:"Delacor_lib_QMH_Enqueue Message (poly).vi"("Message Data"=w110, "Message"="REQ Write DO", "Message Queue in"=w113) -> ("error out"=w107:errorcluster)  [unwired: 7 in, 1 out]
          }
          event User Event {
            # "Another Module called the \"REQ Close DI\" API Method."
            n132 = event-data() -> ("Boolean"=w115:bool)  [unwired: 1 in]
            n133 = Bundle(cluster=T11 {"Boolean"=FALSE} ("REQ Close DI Argument"), "Boolean"=w115) -> (w116:T11)
            n134 = call-poly <vilib>:"Delacor_lib_QMH_Enqueue Message (poly).vi"("Message Data"=w116, "Message"="REQ Close DI", "Message Queue in"=w119) -> ("error out"=w114:errorcluster)  [unwired: 7 in, 1 out]
          }
          event User Event {
            # "Another Module called the \"REQ Close DO\" API Method."
            n135 = event-data() -> ("Boolean"=w121:bool)  [unwired: 1 in]
            n136 = Bundle(cluster=T12 {"Boolean"=FALSE} ("REQ Close DO Argument"), "Boolean"=w121) -> (w122:T12)
            n137 = call-poly <vilib>:"Delacor_lib_QMH_Enqueue Message (poly).vi"("Message Data"=w122, "Message"="REQ Close DO", "Message Queue in"=w125) -> ("error out"=w120:errorcluster)  [unwired: 7 in, 1 out]
          }
          event User Event {
            # "Another Module called the \"REQ Acq DI\" API Method."
            n138 = event-data() -> ("Acq DI"=w127:bool)  [unwired: 1 in]
            n139 = Bundle(cluster=T13 {"Acq DI"=FALSE} ("REQ Acq DI Argument"), "Acq DI"=w127) -> (w128:T13)
            n140 = call-poly <vilib>:"Delacor_lib_QMH_Enqueue Message (poly).vi"("Message Data"=w128, "Message"="REQ Acq DI", "Message Queue in"=w131) -> ("error out"=w126:errorcluster)  [unwired: 7 in, 1 out]
          }
        }
        n141 = call-dynamic "Delacor_lib_QMH_Error Handler - Event Handling Loop.vi"("error in"=w41, "Message Queue in"=w35) -> ("dup error in"=w40:errorcluster)  [unwired: 8 in, 1 out]
      }
    }
    frame Error {
      # "Synchronize Caller Events.vi will inform Start Module.vi that the module has launched and will let the code calling Start Module.vi register for broadcasts and would permit the caller receive the broadcast that an error occurred at launch time."
      n142 = call-dynamic "Delacor_lib_QMH_Release Message Queue.vi"("error in"=w327, "Message Queue"=w325) -> ("error out"=w326:errorcluster)  [unwired: 9 in]
      n143 = call "Synchronize Caller Events.vi"("Singleton Module Admin in"=w328) -> ("error out"=w333:errorcluster)  [unwired: 9 in, 1 out]
      n144 = call "Module Name--constant.vi"() -> ("Module Name"=w331:string)  [unwired: 11 in]
      n145 = Format Into String(format string="An error occurred during initialization. %s is no longer running.", w331) -> (resulting string=w329:string)  [unwired: 2 in, 1 out]
      n146 = Merge Errors(w326, w333) -> (w334:errorcluster)
      n147 = call "Error Reported.vi"("Additional Information"=w329, "Error"=w334) -> ()  [unwired: 9 in, 1 out]
    }
  }
  n148 = while {
    tunnel: w7 -> [w343]
    tunnel: w6 -> [w342]
    shift-right: [w341] -> _
    shift-left: -1 -> [w335]
    shift-right: [w338] -> _
    shift-left: w4 -> [w339]
    tunnel: [w337] -> w2
    tunnel: "DAQ Type" -> [w336]
    stop <- w340 stop-if-true
    # "Acquire DI"
    n149 = event shown="[0] Timeout" {
      selector: w343 -> [_ _ _]
      dyn-events: _ -> [_ _ _]
      timeout: w335 -> [w344 _ w371]
      tunnel: w342 -> [w348 _ _]
      tunnel: [w344 w367 w371] -> w341
      tunnel: [_ _ w372] -> w340
      tunnel: w339 -> [w349 w366 _]
      tunnel: [w347 w366 _] -> w338
      tunnel: [w346 _ _] -> w337
      tunnel: w336 -> [w345 _ _]
      event Timeout {
        n150 = event-data() -> ()  [unwired: 1 in, 1 out]
        n151 = case shown="No Error" w348 {
          selector: w348 -> [w357 w365]
          tunnel: w349 -> [w356 w363]
          tunnel: [w354 w361] -> w347
          tunnel: [w351 w364] -> w346
          tunnel: w345 -> [_ w359]
          frame No Error {
            n152 = Unbundle By Name(w356) -> ("Abstract.lvclass"=w355:refnum<class "Abstract.lvclass">)
            n153 = call-dynamic "Acquire DI.vi"("error in (no error)"=w357, "Abstract in"=w355) -> ("error out"=w352:errorcluster, "Acq DI"=w350:bool[], "Abstract out"=w353:refnum<class "Abstract.lvclass">)  [unwired: 7 in]
            n154 = Bundle By Name(cluster=w356, "Abstract.lvclass"=w353) -> (w354:T3)
            n155 = call "REQ Broadcast DI.vi"("error in"=w352, "Acquire DI"=w350) -> ("error out"=w351:errorcluster)  [unwired: 9 in]
          }
          frame Error {
            n156 = Unbundle By Name(w363) -> ("Abstract.lvclass"=w362:refnum<class "Abstract.lvclass">)
            n157 = local read "DI  Setting"() -> (w358:T2)
            n158 = call-dynamic "Initialize DI.vi"("error in (no error)"=w365, "DI Channel Setting"=w358, "DAQ Type"=w359, "Abstract in"=w362) -> ("error out"=w364:errorcluster, "Abstract out"=w360:refnum<class "Abstract.lvclass">)  [unwired: 6 in]
            n159 = Bundle By Name(cluster=w363, "Abstract.lvclass"=w360) -> (w361:T3)
          }
        }
      }
      event "Acquire DI ?": Value Change {
        n160 = event-data() -> ()  [unwired: 1 in, 1 out]
        n161 = Select(t=0, s="Acquire DI ?", f=-1) -> (s? t:f=w367:i32)
      }
      event User Event {
        n162 = event-data() -> ("Wait for Module to stop?"=w372:bool)  [unwired: 1 in]
      }
    }
  }
  n163 = Merge Errors(w3, w24, w2) -> (w21:errorcluster)
  n164 = call "Close Module.vi"("error in (no error)"=w21, "Module Admin in"=w16) -> ("error out"=w22:errorcluster, "External Launch"=w10:bool, "Module Admin out"=w11:refnum<class "Delacor_lib_QMH_Module Admin.lvclass">)  [unwired: 7 in]
  n165 = Unregister For Events(event registration refnum=w15, error in=w22) -> (error out=w20:errorcluster)
  "error out" <- w20
  n166 = case "External Launch?" shown="True" w10 {
    tunnel: w20 -> [_ w373]
    frame False {
    }
    frame True {
      n167 = case shown="No Error" w373 {
        frame No Error {
          n168 = invoke class="VI" method="FP.Close"() -> ()  [unwired: 3 in, 3 out]
        }
        frame Error {
          n169 = invoke class="VI" method="FP.Open"("Activate"=TRUE ("Activate?")) -> ()  [unwired: 4 in, 5 out]
        }
      }
    }
  }
  n170 = local write "Module Admin"(w11) -> ()
